vi "WILT.vi"() -> ()   [LabVIEW 2016]
uses:
  Type Definitions/WILT Station Test State Cluster.ctl
  Type Definitions/WILT Dryer Test State.ctl
  Type Definitions/WILT Dryer.ctl
  Type Definitions/WILT Dryer Details.ctl
  Type Definitions/WILT Agilent Channel Definition.ctl
  Type Definitions/WILT DAQ Data.ctl
  Type Definitions/WILT Day Night Cycle Enum.ctl
  Type Definitions/WILT Injection Times.ctl
  Type Definitions/WILT Water Injection Control.ctl
  Utility/Save File/File Setup (Public)/Type Definition/Save File DOE File Path Control.ctl
  Utility/Save File/File Setup (Public)/Type Definition/Save File DOE Data Save Filepaths.ctl
  Type Definitions/WILT Agilent Data Cluster.ctl
  Type Definitions/WILT Summary Data.ctl
  Type Definitions/WILT Water Valve Cluster.ctl
  Type Definitions/WILT Start Button Cluster.ctl
  Type Definitions/WILT Water Valve Test Type.ctl
  Utility/Save File/File Setup (Public)/Type Definition/Save File DOE LabView Program.ctl
  Type Definitions/WILT Switch Search.ctl
  Utility/Save File/Public/Type Definitions/Save File FileName Control.ctl
  <vilib>/Utility/file.llb/Write Delimited Spreadsheet (string).vi
  Globals/WILT Globals Main Program.vi
  Utility/Save File/Save File.lvlib
  Utility/Save File/File Setup.lvlib
panel:
  in  "Final Start Presses":i32=1
  in  "Delay After Cutout (Sec)":dbl=5.0 format="%#_13g"
  out "Agilent Semaphore":T1[](array[typedef])
  out "Version":string
  in  "Agilent Switches":T2[](array[typedef])
  in  "Station Timeout Values (1-56) Seconds":dbl[](array[numeric])
  out "Aisle 4 Location":i32
  out "Aisle 4 Update":T3 {"Night Cycle Count" format="%04d"; "Day Cycle Count" format="%04d"}
  out "Aisle 3 Location":i32
  out "Aisle 3 Update":T3 {"Night Cycle Count" format="%04d"; "Day Cycle Count" format="%04d"}
  out "Aisle 2 Location":i32
  out "Aisle 2 Update":T3 {"Night Cycle Count" format="%04d"; "Day Cycle Count" format="%04d"}
  out "Aisle 1A Location":i32
  out "Aisle 1A Update":T3 {"Night Cycle Count" format="%04d"; "Day Cycle Count" format="%04d"}
  out "Aisle 1 Location":i32
  out "Aisle 1 Update":T3 {"Night Cycle Count" format="%04d"; "Day Cycle Count" format="%04d"}
  out "File Refnums":refnum<file>[](array[refnum])
  out "Agilent Data Out":T6
  in  "Save Rate (Seconds)":i32=1
  in  "Scan Rate (Seconds)":i32=1
  out "New File":bool[](array[boolean])
  out "Waiting For Start":u32(colorbox)=15698688
  out "Watering":u32(colorbox)=15698688
  out "No Com":u32(colorbox)
  out "Running":u32(colorbox)=6618880
  out "Stopped":u32(colorbox)=16776960
  out "Fault":u32(colorbox)=16711680
  out "Unused":u32(colorbox)=7171459
  in  "Debug Tab":enum32{"Page 1", "Page 2", "Page 3"}(tab)
  in  "Reset Start Retry All True":bool
  out "Test State array 2":string[](array[string])
  out "Test State array 3":string[](array[string])
  out "Error Out":errorcluster
  in  "Error In":errorcluster
  in  "Debug 2":bool
  out "Test State array 4":string[](array[string])
  out "UI Runs":i32
  in  "Current Threshold":dbl=0.5 format="%#_13g"
  out "Enable Start Retry Array":bool[](array[boolean])
  out "Agilent Switches Locations":T2[](array[typedef])
  out "Send Restart Every? (Sec)":dbl
  out "Station Test State Cluster 2":T7
  out "Previous Run Statistics":T9[](array[typedef])
  in  "Drying Time (Min)":dbl[](array[numeric])
  out "Uncorrected Agilent Data":dbl[](array[numeric])
  out "Corrected Agilent Data":dbl[](array[numeric])
  out "Exit Signal":bool
  in  "Main Tab":T10(tab)
  in  "Shutdown All Valves":bool
  in  "Reset Start Retry":bool
  in  "Day/Night Cycle":T11
  in  "GUI Aisle 3.":T3[](array[typedef]) {"Night Cycle Count" format="%04d"; "Day Cycle Count" format="%04d"}
  in  "GUI Aisle 1 (SLAT).":T3[](array[typedef]) {"Night Cycle Count" format="%04d"; "Day Cycle Count" format="%04d"}
  in  "GUI Aisle 1A (SLAT).":T3[](array[typedef]) {"Night Cycle Count" format="%04d"; "Day Cycle Count" format="%04d"}
  in  "GUI Aisle 2.":T3[](array[typedef]) {"Night Cycle Count" format="%04d"; "Day Cycle Count" format="%04d"}
  in  "GUI Aisle 4.":T3[](array[typedef]) {"Night Cycle Count" format="%04d"; "Day Cycle Count" format="%04d"}
  in  "ExitProg":bool
  in  "Disable Flood Check":bool
  in  "Valve ON Time (mS)":u32=1000
  in  "Number of ON/OFF Cycles":i32=1
  in  "Test Type":T12
  in  "Start Buttons Cluster":T13
  in  "Water Valves Cluster":T14
  in  "Injection Times":T15
  in  "Agilent Refs":refnum<visa-resource-name>[](array[refnum])=["AGILENT1", "AGILENT2", "AGILENT3", "AGILENT4", "AGILENT5", "AGILENT6", "AGILENT7"]
  out "Initialization Complete":bool
  out "Data Out Array":T6
  in  "File Locations":T17[](array[typedef])
  in  "Station Test State Cluster":T7
  out "Elapsed Time.":dbl format="%<%H:%M:%S>t"
  out "4":T1
  out "3":T1
  out "2":T1
  out "1A":T1
  out "1":T1
  # "Dryer Life Test (WILT)"
  # "Day"
  # "Night"
  # "Day"
  # "Night"
  # "Day"
  # "Night"
  # "Day"
  # "Night"
  # "Day"
  # "Night"
  # "Day"
  # "Night"
  # "Day"
  # "Night"
  # "Day"
  # "Night"
  # "Day"
  # "Night"
  # "Day"
  # "Night"
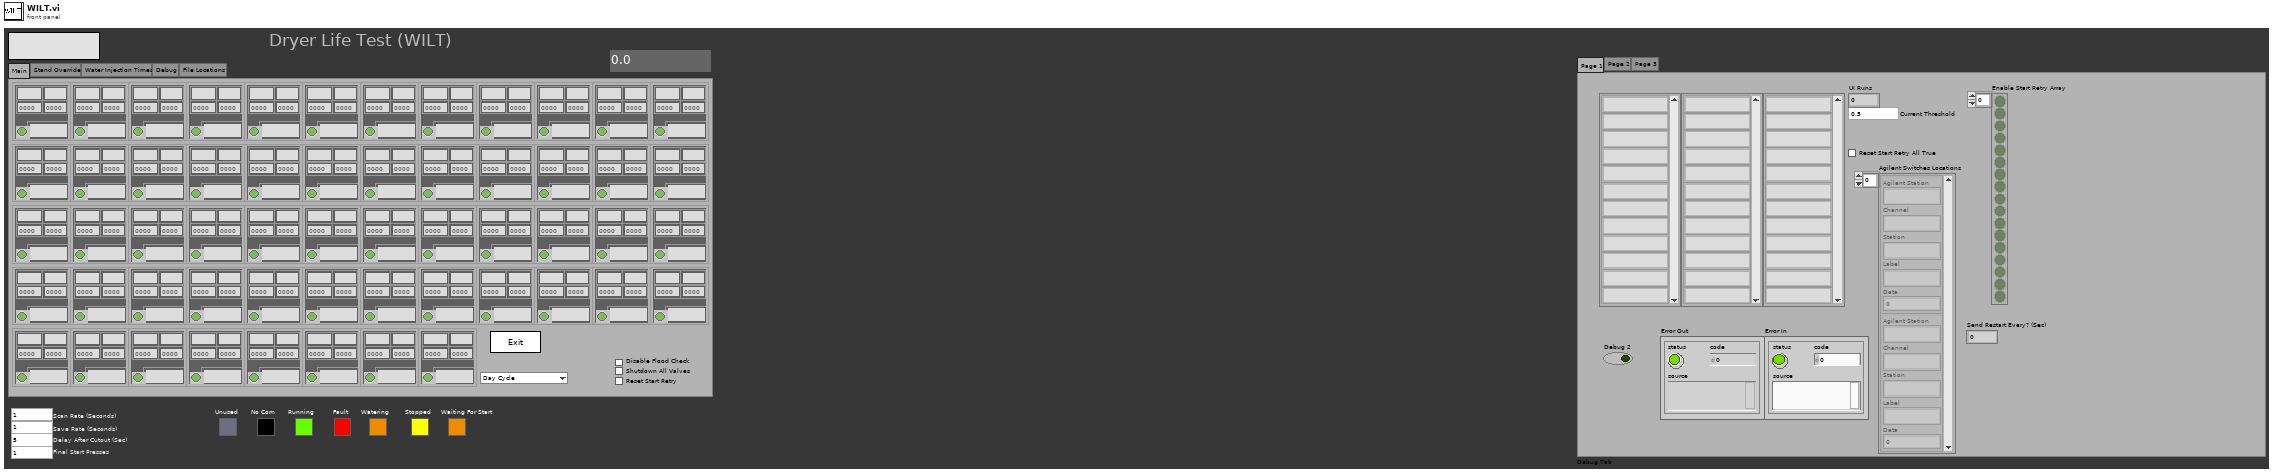
[diagram p1: front panel]
types:
  T1 = typedef "Semaphore RefNum" = refnum<k1>
  T2 = typedef "WILT Agilent Channel Definition.ctl" = cluster{"Channel":string, "Station":string, "Label":string, "Agilent Station":string, "Data":dbl}
  T3 = typedef "WILT Dryer.ctl" = cluster{"Lab ID":string, "Day Cycle Count":i32, "Station Label":string, "Dryer Details":T4, "Status Color":u32, "Invisible Button":bool, "Night Cycle Count":i32, "Station Index":i32, "Cycle Index":string, "Audit Alert":bool, "Agilent Channel Definition":T2, "DAQ Data":T5}
  T4 = typedef "WILT Dryer Details.ctl" = cluster{"Station":string, "Lab ID":string, "TR Number":string}
  T5 = typedef "WILT DAQ Data.ctl" = cluster{"L1 Current":dbl, "L2 Current":dbl, "Temperature  Deg F (TC)":dbl, "Volts":dbl, "Volts (208)":dbl, "SW (208)":dbl}
  T6 = typedef "WILT Agilent Data Cluster.ctl" = T2[]
  T7 = typedef "WILT Station Test State Cluster.ctl" = cluster{"Station Test State 1":T8, "Station Test State 2":T8, "Station Test State 3":T8, "Station Test State 4":T8, "Station Test State 5":T8, "Station Test State 6":T8, "Station Test State 7":T8, "Station Test State 8":T8, "Station Test State 9":T8, "Station Test State 10":T8, "Station Test State 11":T8, "Station Test State 12":T8, "Station Test State 13":T8, "Station Test State 14":T8, "Station Test State 15":T8, "Station Test State 16":T8, "Station Test State 17":T8, "Station Test State 18":T8, "Station Test State 19":T8, "Station Test State 20":T8, "Station Test State 21":T8, "Station Test State 22":T8, "Station Test State 23":T8, "Station Test State 24":T8, "Station Test State 25":T8, "Station Test State 26":T8, "Station Test State 27":T8, "Station Test State 28":T8, "Station Test State 29":T8, "Station Test State 30":T8, "Station Test State 31":T8, "Station Test State 32":T8, "Station Test State 33":T8, "Station Test State 34":T8, "Station Test State 35":T8, "Station Test State 36":T8, "Station Test State 37":T8, "Station Test State 38":T8, "Station Test State 39":T8, "Station Test State 40":T8, "Station Test State 41":T8, "Station Test State 42":T8, "Station Test State 43":T8, "Station Test State 44":T8, "Station Test State 45":T8, "Station Test State 46":T8, "Station Test State 47":T8, "Station Test State 48":T8, "Station Test State 49":T8, "Station Test State 50":T8, "Station Test State 51":T8, "Station Test State 52":T8, "Station Test State 53":T8, "Station Test State 54":T8, "Station Test State 55":T8, "Station Test State 56":T8}
  T8 = typedef "WILT Dryer Test State.ctl" = enum16{"No Serial Number", "Waiting for Dryer To Start", "Drying Clothes", "Water Injection 1 (On)", "Water Injection 1 Timer", "Water Injection 1 (Off)", "Pause Dryer", "Sending Start Stop CMD", "Pause Dryer 2", "Sending Start Stop CMD 2", "Drying Clothes 2", "Water Injection 2 (On)", "Water Injection 2 Timer", "Water Injection 2 (Off)", "Drying Clothes 3", "Cooling Down", "Sending Start Stop CMD 3", "Increment Cycle"}
  T9 = typedef "WILT Summary Data.ctl" = cluster{"Cycle Time (Minutes)":dbl, "L1 Current (Amps)":dbl, "L2 Current (Amps)":dbl, "TC Temperature (Deg F)":dbl, "Voltage (Volts)":dbl, "Voltage-208 (Volts)":dbl, "208V Switch (Ohms)":dbl, "Cycle Number":i32}
  T10 = enum32{"Main", "Stand Override", "Water Injection Times", "Debug", "File Locations"}
  T11 = typedef "WILT Day Night Cycle Enum.ctl" = enum16{"Day Cycle", "Night Cycle", "Day Cycle (No Water)"}
  T12 = typedef "WILT Water Valve Test Type.ctl" = enum16{"Cycle Valve Control", "Full Valve Control"}
  T13 = typedef "WILT Start Button Cluster.ctl" = cluster{"Start Button 21":bool, "Start Button 22":bool, "Start Button 23":bool, "Start Button 24":bool, "Start Button 25":bool, "Start Button 26":bool, "Start Button 27":bool, "Start Button 28":bool, "Start Button 29":bool, "Start Button 30":bool, "Start Button 31":bool, "Start Button 32":bool, "Start Button 33":bool, "Start Button 34":bool, "Start Button 35":bool, "Start Button 36":bool, "Start Button 37":bool, "Start Button 38":bool, "Start Button 39":bool, "Start Button 40":bool, "Start Button 41":bool, "Start Button 42":bool, "Start Button 43":bool, "Start Button 44":bool, "Start Button 12":bool, "Start Button 11":bool, "Start Button 10":bool, "Start Button 9":bool, "Start Button 8":bool, "Start Button 7":bool, "Start Button 6":bool, "Start Button 5":bool, "Start Button 4":bool, "Start Button 3":bool, "Start Button 2":bool, "Start Button 1":bool, "Start Button 20":bool, "Start Button 19":bool, "Start Button 18":bool, "Start Button 17":bool, "Start Button 16":bool, "Start Button 15":bool, "Start Button 14":bool, "Start Button 13":bool, "Start Button 45":bool, "Start Button 46":bool, "Start Button 47":bool, "Start Button 48":bool, "Start Button 49":bool, "Start Button 50":bool, "Start Button 51":bool, "Start Button 52":bool, "Start Button 53":bool, "Start Button 54":bool, "Start Button 55":bool, "Start Button 56":bool}
  T14 = typedef "WILT Water Valve Cluster.ctl" = cluster{"Valve 1":bool, "Valve 2":bool, "Valve 3":bool, "Valve 4":bool, "Valve 5":bool, "Valve 6":bool, "Valve 7":bool, "Valve 8":bool, "Valve 9":bool, "Valve 10":bool, "Valve 11":bool, "Valve 12":bool, "Valve 13":bool, "Valve 14":bool, "Valve 15":bool, "Valve 16":bool, "Valve 17":bool, "Valve 18":bool, "Valve 19":bool, "Valve 20":bool, "Valve 21":bool, "Valve 22":bool, "Valve 23":bool, "Valve 24":bool, "Valve 25":bool, "Valve 26":bool, "Valve 27":bool, "Valve 28":bool, "Valve 29":bool, "Valve 30":bool, "Valve 31":bool, "Valve 32":bool, "Valve 33":bool, "Valve 34":bool, "Valve 35":bool, "Valve 36":bool, "Valve 37":bool, "Valve 38":bool, "Valve 39":bool, "Valve 40":bool, "Valve 41":bool, "Valve 42":bool, "Valve 43":bool, "Valve 44":bool, "Valve 45":bool, "Valve 46":bool, "Valve 47":bool, "Valve 48":bool, "Valve 49":bool, "Valve 50":bool, "Valve 51":bool, "Valve 52":bool, "Valve 53":bool, "Valve 54":bool, "Valve 55":bool, "Valve 56":bool}
  T15 = typedef "WILT Injection Times.ctl" = T16[]
  T16 = typedef "WILT Water Injection Control.ctl" = cluster{"Injection 1 (Seconds)":dbl, "Injection 2 (Seconds)":dbl}
  T17 = typedef "File Setup.lvlib/Save File DOE File Path Control.ctl" = cluster{"General Setup Paths":cluster{"Calibration File Path":path, "DOE Capacity Path":path, "Data Folder Path":path, "RLT Backup Data Path":path, "Tool Base Path":path, "General Startup Config Path":path, "File Save Previous Run Path":path, "File Save Configuration Data Path":path}, "Data File Paths":T18, "New Summary Created":bool, "Check Location Interval (Second)":i32}
  T18 = typedef "File Setup.lvlib/Save File DOE Data Save Filepaths.ctl" = cluster{"Data File Path":path, "Debug File Path":path, "Bus Log Path":path, "Current":path, "Summary":path}
  T19 = typedef "WILT Switch Search.ctl" = string
  T20 = enum32{"invalid app kind", "Development System", "Run Time System", "Student Edition", "Embedded LabVIEW", "Evaluation", "Custom"}
  T21 = typedef "Save File.lvlib/Save File FileName Control.ctl" = cluster{"Debug File DIR":string, "Inverter And MC File DIR":string}
  T22 = enum32{"Invalid", "Standard", "Closed", "Hidden", "Minimized", "Maximized"}
  T23 = typedef "File Setup.lvlib/Save File DOE LabView Program.ctl" = enum16{"No Name Found", "DOE Stand", "Dishwasher Kitchen", "Portable Stand", "HEWH", "Dryer", "Dryer WILT", "HCC", "PRAT", "HEWH RLT", "Refrigeration"}
  T24 = cluster{"Send Restart Every? (Sec)":dbl, "Enable Start Retry Array":bool[], "Agilent Switches":T2[], "States":string, "Core":cluster{"Current VI Reference":refnum<vi>, "Close Panel on Exit?":bool}, "Station Test State Cluster":T7, "GUI Aisle 4.":T3[], "GUI Aisle 3.":T3[], "GUI Aisle 2.":T3[], "GUI Aisle 1A (SLAT).":T3[], "GUI Aisle 1 (SLAT).":T3[], "Agilent Refs":refnum<visa-resource-name>[], "Configuration Startup Directorys":T21, "File Locations":T17[], "Day/Night Cycle Input":T11, "Injection Times Input":T15, "Current Threshold":dbl, "Station Timeout Values (1-56) Seconds":dbl[], "Drying Time (Min)":dbl[]}
  T25 = cluster{"Current VI Reference":refnum<vi>, "Close Panel on Exit?":bool}
  T26 = typedef "Save File.lvlib/Save File Washer.ctl" = cluster{"Appliance Details":T27, "Display Data (RLT)":T33}
  T27 = typedef "File Setup.lvlib/Save File DISH Dishwasher Details.ctl" = cluster{"FileVersionInfo":T28, "Dishwasher Info":cluster{"Open Cup Weight (gm):":dbl, "Auto Cup Weight (gm):":dbl, "Detergent-Dish:":string, "Inlet Temperature-Dish:":string, "Cycle Mode-Dish:":string, "Unit Control-Dish:":string, "Manufacturer-Dish:":string}, "Washer Info":cluster{"Hot Water Temperature (Fahrenheit):":string, "Cold Water Temperature (Fahrenheit):":string, "Capacity (cu.ft):":dbl, "Initial Cloth Weight:":dbl, "Cloth Lot:":i32, "Model Family:":string, "Program Name:":string, "Cycle Selection:":string, "Wash Temperature:":string, "Rinse Temperature:":string, "Load Size:":string}, "File Name Output Array":string[][], "Calibration Output Array":string[][], "Appliance Common":T29, "Water Heater":cluster{"Heating Mode:":string}, "Dryer":cluster{"Heat Setting:":T30, "Washer Water Temperature (60 ± 5°F):":u16, "Water Hardness (PPM):":u16, "Dryness Setting:":T30, "Dryer Type:":string, "Exhaust:":string, "Drying Cycle:":string, "Load Type:":string, "Nominal Load Weight":string, "Dryer Initial IMC Data":T31}}
  T28 = typedef "FileVersionInformation.ctl" = cluster{"FileVersion":string, "ProductName":string, "InternalName":string, "CompanyName":string, "LegalCopyright":string, "FileDescription":string}
  T29 = typedef "DOE Appliance Common.ctl" = cluster{"Engineer:":string, "Model Number:":string, "Serial Number:":string, "Comments:":string, "Station ID:":string, "Technician:":string, "TR Number:":string, "Lab ID:":string, "Voltage:":string, "Water Pressure (PSI):":string, "Test Date:":string, "Computer Name:":string, "IP Address:":string, "Ambient RH:":string, "Frequency:":string, "Build:":string, "Filename:":string, "Test Type:":string, "Load Run #:":i32, "Ambient Temperature (F):":string, "File Path:":path, "Cycles Per Year":u32}
  T30 = typedef "Custom Pallet String.ctl" = string
  T31 = typedef "DPT IMC Data.ctl" = cluster{"Measured IMC (lbs)":dbl, "Actual Initial RMC (%)":dbl, "RMC (Desired %)":dbl, "Bone Dry Wt(lbs)":dbl, "Tolerance(%)":dbl, "Actual Final RMC (%)":dbl, "CEF (lbf/kWh)":dbl, "Minimum Weight (lbf)":dbl, "Average Weight (lbf)":dbl, "Maximum Weight (lbf)":dbl, "Measured IMC In Range?":bool, "Moisture Reduction Factor":dbl, "Field Use Factor":dbl, "Empty Dryer Cold Weigth":dbl, "Energy Standard":T32, "Weight Cloth (lbs)":dbl, "Relative Moisture Content (%)":dbl, "Relative Moisture Content - Avg (%)":dbl}
  T32 = typedef "DOE Dryer Standard.ctl" = enum16{"D2-Automatic Dryer", "D2-Timer Dryer", "D1-Automatic Dryer", "D1-Timer Dryer", "Other"}
  T33 = typedef "Save File Appliance Display.ctl" = cluster{"Status Color":u32, "Serial Number Display":string, "Cycle Count Display":i32, "Station Label Display":string, "Current Run Start Time Display":dbl, "Board ID Display":string, "RPM Display":u32, "Current Display":dbl, "Current Path Display":path, "Saving Display":bool, "Unit Type Display":T34, "Total Time On Display":dbl, "UI Button":bool}
  T34 = typedef "Save File.lvlib/Save File Unit Type.ctl" = enum32{"", "Viper", "Hawk", "2015"}
  T35 = cluster{"Core":cluster{"Current VI Reference":refnum<vi>, "Close Panel on Exit?":bool}, "Agilent Refs":refnum<visa-resource-name>[], "Data Out Array":T6}
  T36 = cluster{"Core":cluster{"Current VI Reference":refnum<vi>, "Close Panel on Exit?":bool}, "First Time Through?":bool[], "File Locations":T17[], "File Refnums":refnum<file>[]}
  T37 = cluster{"File Locations":T17[], "WILT Summary Array":T9[], "Units To Process":bool[]}
  T38 = cluster{"Your Boolean data":bool, "Your string data":string}
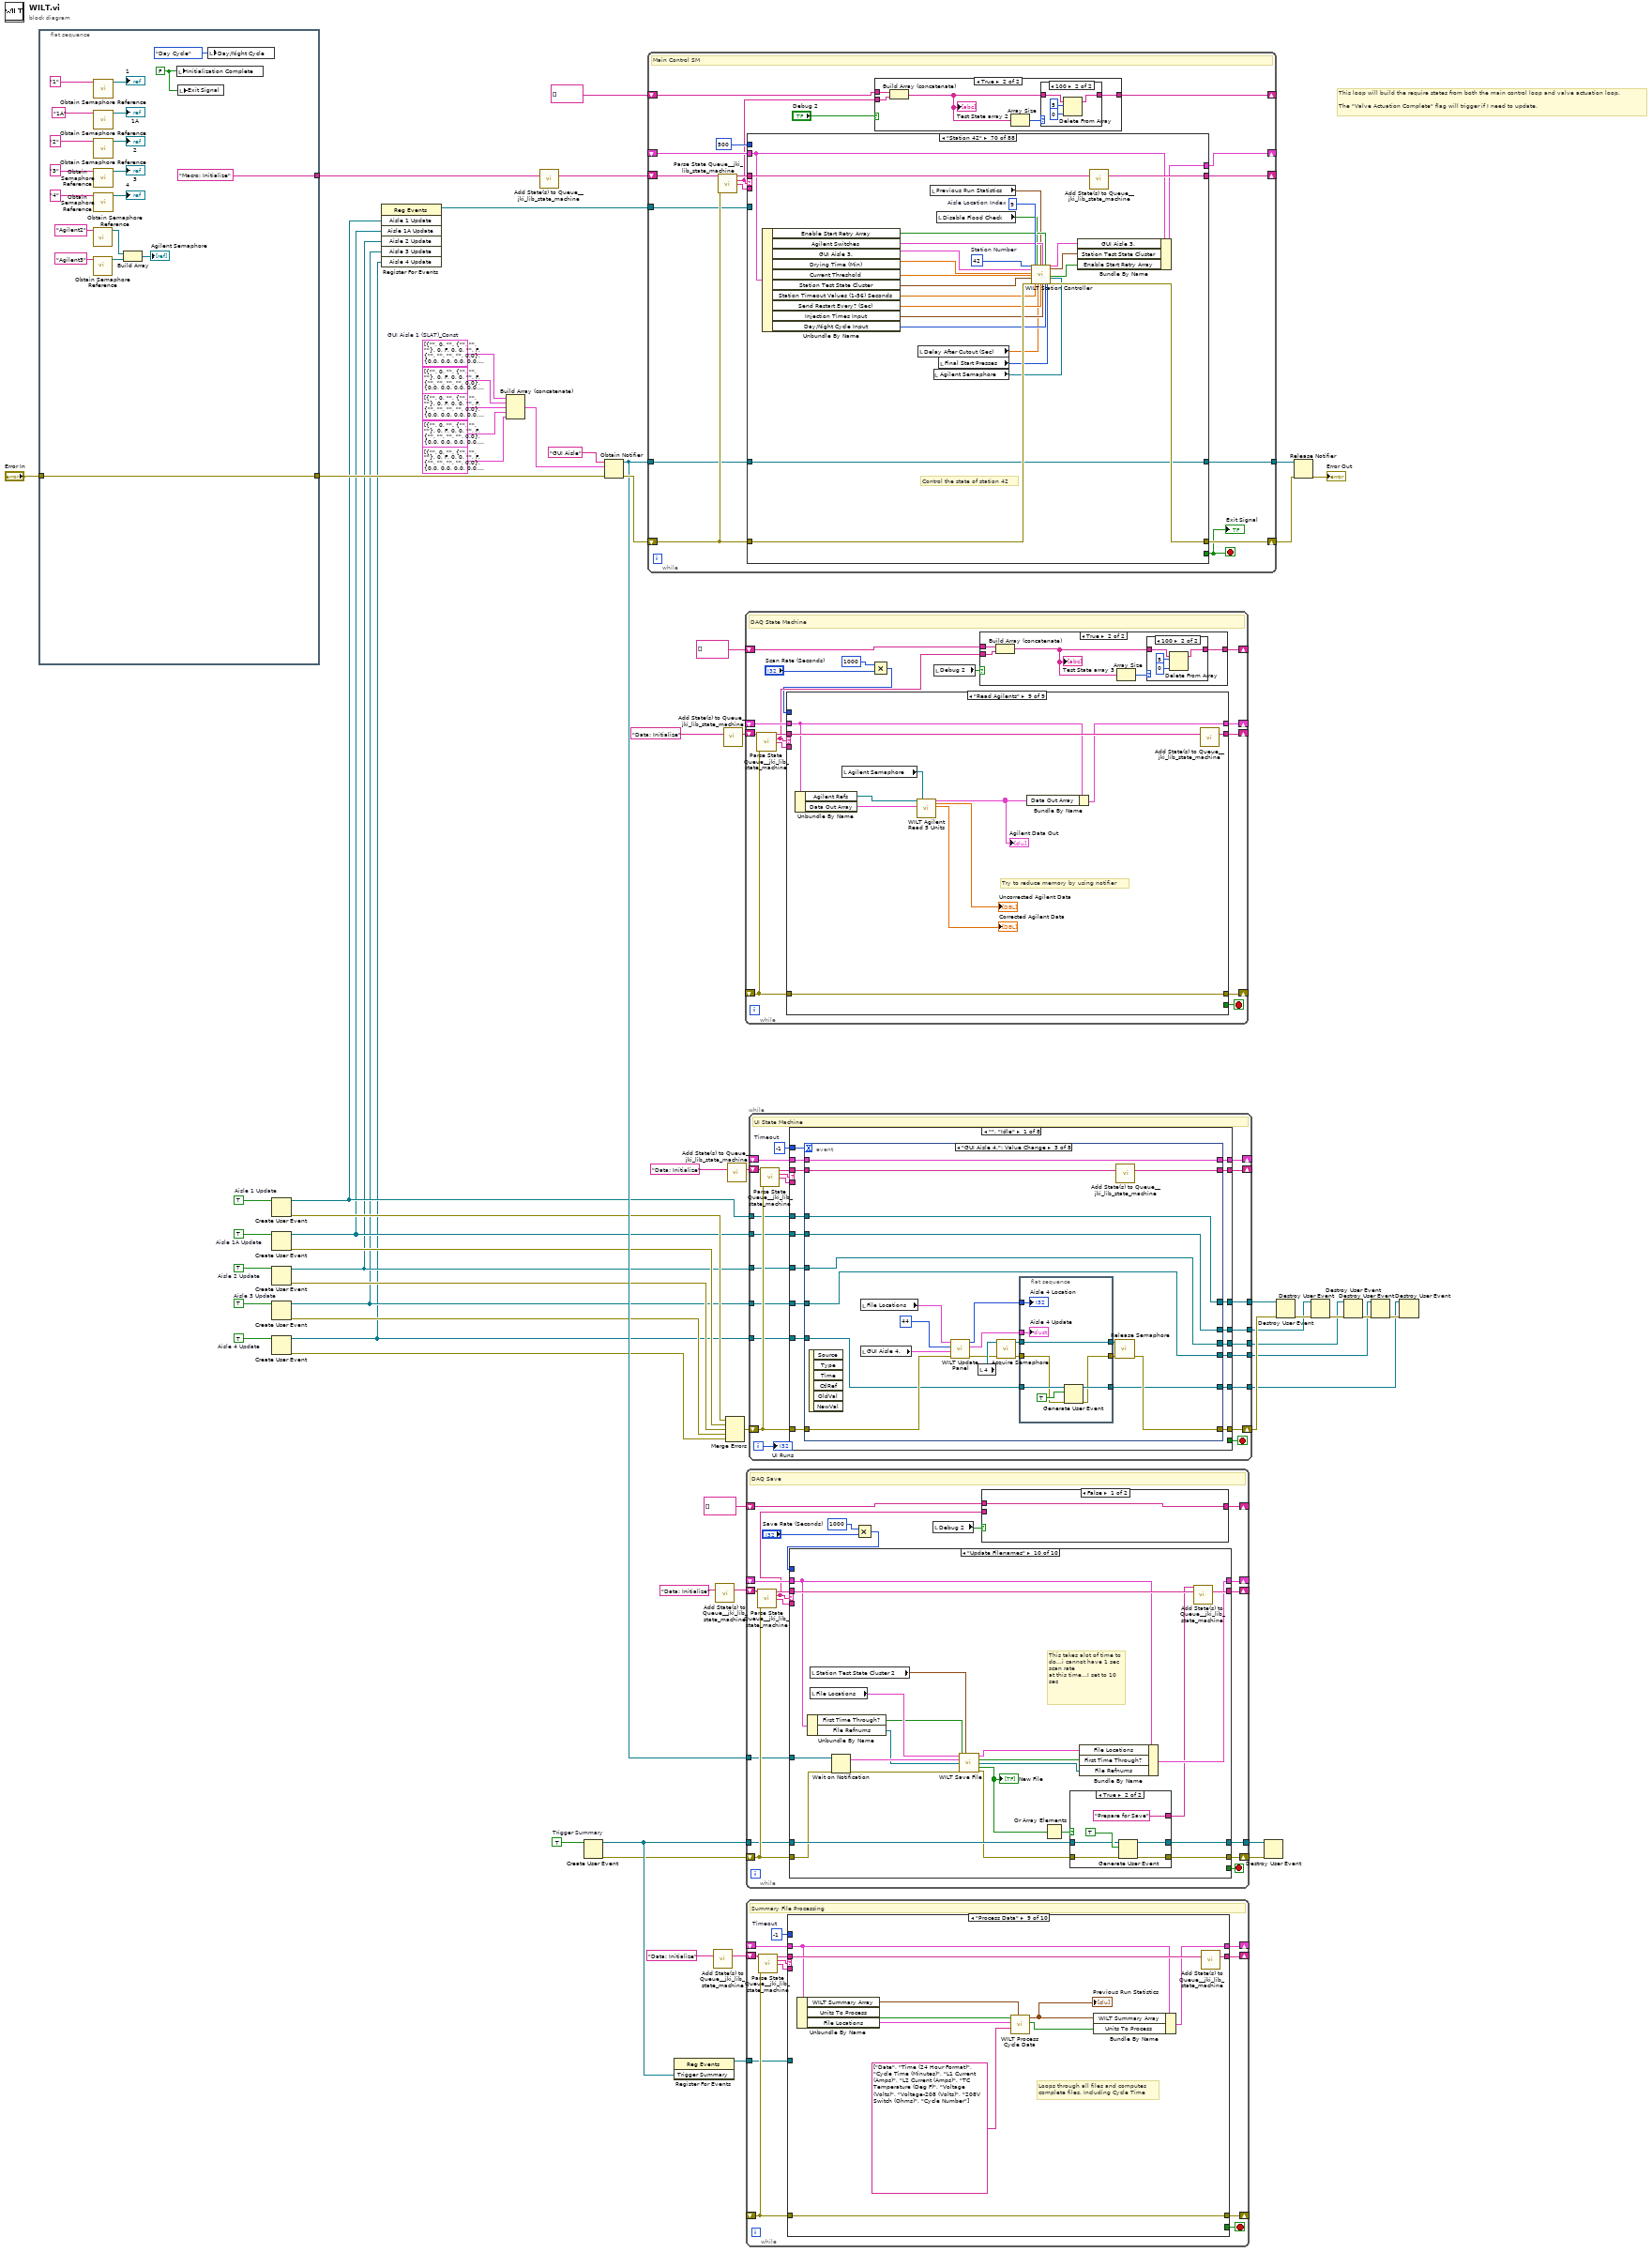
[diagram p0: block diagram]
diagram:
  w24 = TRUE  # Aisle 4 Update
  w25 = TRUE  # Aisle 3 Update
  w26 = TRUE  # Aisle 2 Update
  w27 = TRUE  # Aisle 1A Update
  w28 = TRUE  # Aisle 1 Update
  w39 = T3[] [{"Lab ID"="", "Day Cycle Count"=0, "Station Label"="", "Dryer Details"={"Station"="", "Lab ID"="", "TR Number"=""}, "Status Color"=0, "Invisible Button"=FALSE, "Night Cycle Count"=0, "Station Index"=0, "Cycle Index"="", "Audit Alert"=FALSE, "Agilent Channel Definition"={"Channel"="", "Station"="", "Label"="", "Agilent Station"="", "Data"=0.0}, "DAQ Data"={"L1 Current"=0.0, "L2 Current"=0.0, "Temperature  Deg F (TC)"=0.0, "Volts"=0.0, "Volts (208)"=0.0, "SW (208)"=0.0}}, {"Lab ID"="", "Day Cycle Count"=0, "Station Label"="", "Dryer Details"={"Station"="", "Lab ID"="", "TR Number"=""}, "Status Color"=0, "Invisible Button"=FALSE, "Night Cycle Count"=0, "Station Index"=0, "Cycle Index"="", "Audit Alert"=FALSE, "Agilent Channel Definition"={"Channel"="", "Station"="", "Label"="", "Agilent Station"="", "Data"=0.0}, "DAQ Data"={"L1 Current"=0.0, "L2 Current"=0.0, "Temperature  Deg F (TC)"=0.0, "Volts"=0.0, "Volts (208)"=0.0, "SW (208)"=0.0}}, {"Lab ID"="", "Day Cycle Count"=0, "Station Label"="", "Dryer Details"={"Station"="", "Lab ID"="", "TR Number"=""}, "Status Color"=0, "Invisible Button"=FALSE, "Night Cycle Count"=0, "Station Index"=0, "Cycle Index"="", "Audit Alert"=FALSE, "Agilent Channel Definition"={"Channel"="", "Station"="", "Label"="", "Agilent Station"="", "Data"=0.0}, "DAQ Data"={"L1 Current"=0.0, "L2 Current"=0.0, "Temperature  Deg F (TC)"=0.0, "Volts"=0.0, "Volts (208)"=0.0, "SW (208)"=0.0}}, {"Lab ID"="", "Day Cycle Count"=0, "Station Label"="", "Dryer Details"={"Station"="", "Lab ID"="", "TR Number"=""}, "Status Color"=0, "Invisible Button"=FALSE, "Night Cycle Count"=0, "Station Index"=0, "Cycle Index"="", "Audit Alert"=FALSE, "Agilent Channel Definition"={"Channel"="", "Station"="", "Label"="", "Agilent Station"="", "Data"=0.0}, "DAQ Data"={"L1 Current"=0.0, "L2 Current"=0.0, "Temperature  Deg F (TC)"=0.0, "Volts"=0.0, "Volts (208)"=0.0, "SW (208)"=0.0}}, {"Lab ID"="", "Day Cycle Count"=0, "Station Label"="", "Dryer Details"={"Station"="", "Lab ID"="", "TR Number"=""}, "Status Color"=0, "Invisible Button"=FALSE, "Night Cycle Count"=0, "Station Index"=0, "Cycle Index"="", "Audit Alert"=FALSE, "Agilent Channel Definition"={"Channel"="", "Station"="", "Label"="", "Agilent Station"="", "Data"=0.0}, "DAQ Data"={"L1 Current"=0.0, "L2 Current"=0.0, "Temperature  Deg F (TC)"=0.0, "Volts"=0.0, "Volts (208)"=0.0, "SW (208)"=0.0}}, {"Lab ID"="", "Day Cycle Count"=0, "Station Label"="", "Dryer Details"={"Station"="", "Lab ID"="", "TR Number"=""}, "Status Color"=0, "Invisible Button"=FALSE, "Night Cycle Count"=0, "Station Index"=0, "Cycle Index"="", "Audit Alert"=FALSE, "Agilent Channel Definition"={"Channel"="", "Station"="", "Label"="", "Agilent Station"="", "Data"=0.0}, "DAQ Data"={"L1 Current"=0.0, "L2 Current"=0.0, "Temperature  Deg F (TC)"=0.0, "Volts"=0.0, "Volts (208)"=0.0, "SW (208)"=0.0}}, {"Lab ID"="", "Day Cycle Count"=0, "Station Label"="", "Dryer Details"={"Station"="", "Lab ID"="", "TR Number"=""}, "Status Color"=0, "Invisible Button"=FALSE, "Night Cycle Count"=0, "Station Index"=0, "Cycle Index"="", "Audit Alert"=FALSE, "Agilent Channel Definition"={"Channel"="", "Station"="", "Label"="", "Agilent Station"="", "Data"=0.0}, "DAQ Data"={"L1 Current"=0.0, "L2 Current"=0.0, "Temperature  Deg F (TC)"=0.0, "Volts"=0.0, "Volts (208)"=0.0, "SW (208)"=0.0}}, {"Lab ID"="", "Day Cycle Count"=0, "Station Label"="", "Dryer Details"={"Station"="", "Lab ID"="", "TR Number"=""}, "Status Color"=0, "Invisible Button"=FALSE, "Night Cycle Count"=0, "Station Index"=0, "Cycle Index"="", "Audit Alert"=FALSE, "Agilent Channel Definition"={"Channel"="", "Station"="", "Label"="", "Agilent Station"="", "Data"=0.0}, "DAQ Data"={"L1 Current"=0.0, "L2 Current"=0.0, "Temperature  Deg F (TC)"=0.0, "Volts"=0.0, "Volts (208)"=0.0, "SW (208)"=0.0}}, {"Lab ID"="", "Day Cycle Count"=0, "Station Label"="", "Dryer Details"={"Station"="", "Lab ID"="", "TR Number"=""}, "Status Color"=0, "Invisible Button"=FALSE, "Night Cycle Count"=0, "Station Index"=0, "Cycle Index"="", "Audit Alert"=FALSE, "Agilent Channel Definition"={"Channel"="", "Station"="", "Label"="", "Agilent Station"="", "Data"=0.0}, "DAQ Data"={"L1 Current"=0.0, "L2 Current"=0.0, "Temperature  Deg F (TC)"=0.0, "Volts"=0.0, "Volts (208)"=0.0, "SW (208)"=0.0}}, {"Lab ID"="", "Day Cycle Count"=0, "Station Label"="", "Dryer Details"={"Station"="", "Lab ID"="", "TR Number"=""}, "Status Color"=0, "Invisible Button"=FALSE, "Night Cycle Count"=0, "Station Index"=0, "Cycle Index"="", "Audit Alert"=FALSE, "Agilent Channel Definition"={"Channel"="", "Station"="", "Label"="", "Agilent Station"="", "Data"=0.0}, "DAQ Data"={"L1 Current"=0.0, "L2 Current"=0.0, "Temperature  Deg F (TC)"=0.0, "Volts"=0.0, "Volts (208)"=0.0, "SW (208)"=0.0}}, {"Lab ID"="", "Day Cycle Count"=0, "Station Label"="", "Dryer Details"={"Station"="", "Lab ID"="", "TR Number"=""}, "Status Color"=0, "Invisible Button"=FALSE, "Night Cycle Count"=0, "Station Index"=0, "Cycle Index"="", "Audit Alert"=FALSE, "Agilent Channel Definition"={"Channel"="", "Station"="", "Label"="", "Agilent Station"="", "Data"=0.0}, "DAQ Data"={"L1 Current"=0.0, "L2 Current"=0.0, "Temperature  Deg F (TC)"=0.0, "Volts"=0.0, "Volts (208)"=0.0, "SW (208)"=0.0}}, {"Lab ID"="", "Day Cycle Count"=0, "Station Label"="", "Dryer Details"={"Station"="", "Lab ID"="", "TR Number"=""}, "Status Color"=0, "Invisible Button"=FALSE, "Night Cycle Count"=0, "Station Index"=0, "Cycle Index"="", "Audit Alert"=FALSE, "Agilent Channel Definition"={"Channel"="", "Station"="", "Label"="", "Agilent Station"="", "Data"=0.0}, "DAQ Data"={"L1 Current"=0.0, "L2 Current"=0.0, "Temperature  Deg F (TC)"=0.0, "Volts"=0.0, "Volts (208)"=0.0, "SW (208)"=0.0}}]  # GUI Aisle 1 (SLAT)_Const
  w46 = TRUE  # Trigger Summary
  # "This loop will build the require states from both the main control loop and valve actuation loop.\n\nThe \"Valve Actuation Complete\" flag will trigger if I need to update."
  n1 = flat-sequence {
    tunnel: ["Macro: Initialize"] -> w59
    tunnel: [w76] -> w34
    tunnel: "Error In" -> [w76]
    frame #0 {
      w78 = FALSE ("Initialization Complete")
      n2 = call <vilib>:"Obtain Semaphore Reference.vi"("name (unnamed)"="Agilent2") -> ("semaphore"=w63:T1)  [unwired: 4 in, 2 out]
      n3 = call <vilib>:"Obtain Semaphore Reference.vi"("name (unnamed)"="Agilent3") -> ("semaphore"=w62:T1)  [unwired: 4 in, 2 out]
      n4 = call <vilib>:"Obtain Semaphore Reference.vi"("name (unnamed)"="1") -> ("semaphore"=→"1":T1)  [unwired: 4 in, 2 out]
      n5 = call <vilib>:"Obtain Semaphore Reference.vi"("name (unnamed)"="1A") -> ("semaphore"=→"1A":T1)  [unwired: 4 in, 2 out]
      n6 = call <vilib>:"Obtain Semaphore Reference.vi"("name (unnamed)"="2") -> ("semaphore"=→"2":T1)  [unwired: 4 in, 2 out]
      n7 = call <vilib>:"Obtain Semaphore Reference.vi"("name (unnamed)"="3") -> ("semaphore"=→"3":T1)  [unwired: 4 in, 2 out]
      n8 = call <vilib>:"Obtain Semaphore Reference.vi"("name (unnamed)"="4") -> ("semaphore"=→"4":T1)  [unwired: 4 in, 2 out]
      n9 = Build Array(w63, w62) -> (→"Agilent Semaphore":T1[])
      n10 = local write "Initialization Complete"(w78) -> ()
      n11 = local write "Exit Signal"(w78) -> ()
      n12 = local write "Day/Night Cycle"(WILT_Day_Night_Cycle_Enum."Day Cycle" ("Day/Night Cycle")) -> ()
    }
  }
  n13 = Create User Event(user event datatype=w28) -> (user event=w7:refnum<user-event>, error out=w23:errorcluster)  [unwired: 1 in]
  n14 = Create User Event(user event datatype=w27) -> (user event=w6:refnum<user-event>, error out=w22:errorcluster)  [unwired: 1 in]
  n15 = Create User Event(user event datatype=w26) -> (user event=w5:refnum<user-event>, error out=w21:errorcluster)  [unwired: 1 in]
  n16 = Create User Event(user event datatype=w25) -> (user event=w4:refnum<user-event>, error out=w20:errorcluster)  [unwired: 1 in]
  n17 = Create User Event(user event datatype=w24) -> (user event=w3:refnum<user-event>, error out=w19:errorcluster)  [unwired: 1 in]
  n18 = register-events(w7, w6, w5, w4, w3) -> (reference out=w2:refnum<event-registration>)  [unwired: 2 in, 1 out]
  n19 = Build Array (concatenate)(w39, T3[] [{"Lab ID"="", "Day Cycle Count"=0, "Station Label"="", "Dryer Details"={"Station"="", "Lab ID"="", "TR Number"=""}, "Status Color"=0, "Invisible Button"=FALSE, "Night Cycle Count"=0, "Station Index"=0, "Cycle Index"="", "Audit Alert"=FALSE, "Agilent Channel Definition"={"Channel"="", "Station"="", "Label"="", "Agilent Station"="", "Data"=0.0}, "DAQ Data"={"L1 Current"=0.0, "L2 Current"=0.0, "Temperature  Deg F (TC)"=0.0, "Volts"=0.0, "Volts (208)"=0.0, "SW (208)"=0.0}}, {"Lab ID"="", "Day Cycle Count"=0, "Station Label"="", "Dryer Details"={"Station"="", "Lab ID"="", "TR Number"=""}, "Status Color"=0, "Invisible Button"=FALSE, "Night Cycle Count"=0, "Station Index"=0, "Cycle Index"="", "Audit Alert"=FALSE, "Agilent Channel Definition"={"Channel"="", "Station"="", "Label"="", "Agilent Station"="", "Data"=0.0}, "DAQ Data"={"L1 Current"=0.0, "L2 Current"=0.0, "Temperature  Deg F (TC)"=0.0, "Volts"=0.0, "Volts (208)"=0.0, "SW (208)"=0.0}}, {"Lab ID"="", "Day Cycle Count"=0, "Station Label"="", "Dryer Details"={"Station"="", "Lab ID"="", "TR Number"=""}, "Status Color"=0, "Invisible Button"=FALSE, "Night Cycle Count"=0, "Station Index"=0, "Cycle Index"="", "Audit Alert"=FALSE, "Agilent Channel Definition"={"Channel"="", "Station"="", "Label"="", "Agilent Station"="", "Data"=0.0}, "DAQ Data"={"L1 Current"=0.0, "L2 Current"=0.0, "Temperature  Deg F (TC)"=0.0, "Volts"=0.0, "Volts (208)"=0.0, "SW (208)"=0.0}}, {"Lab ID"="", "Day Cycle Count"=0, "Station Label"="", "Dryer Details"={"Station"="", "Lab ID"="", "TR Number"=""}, "Status Color"=0, "Invisible Button"=FALSE, "Night Cycle Count"=0, "Station Index"=0, "Cycle Index"="", "Audit Alert"=FALSE, "Agilent Channel Definition"={"Channel"="", "Station"="", "Label"="", "Agilent Station"="", "Data"=0.0}, "DAQ Data"={"L1 Current"=0.0, "L2 Current"=0.0, "Temperature  Deg F (TC)"=0.0, "Volts"=0.0, "Volts (208)"=0.0, "SW (208)"=0.0}}, {"Lab ID"="", "Day Cycle Count"=0, "Station Label"="", "Dryer Details"={"Station"="", "Lab ID"="", "TR Number"=""}, "Status Color"=0, "Invisible Button"=FALSE, "Night Cycle Count"=0, "Station Index"=0, "Cycle Index"="", "Audit Alert"=FALSE, "Agilent Channel Definition"={"Channel"="", "Station"="", "Label"="", "Agilent Station"="", "Data"=0.0}, "DAQ Data"={"L1 Current"=0.0, "L2 Current"=0.0, "Temperature  Deg F (TC)"=0.0, "Volts"=0.0, "Volts (208)"=0.0, "SW (208)"=0.0}}, {"Lab ID"="", "Day Cycle Count"=0, "Station Label"="", "Dryer Details"={"Station"="", "Lab ID"="", "TR Number"=""}, "Status Color"=0, "Invisible Button"=FALSE, "Night Cycle Count"=0, "Station Index"=0, "Cycle Index"="", "Audit Alert"=FALSE, "Agilent Channel Definition"={"Channel"="", "Station"="", "Label"="", "Agilent Station"="", "Data"=0.0}, "DAQ Data"={"L1 Current"=0.0, "L2 Current"=0.0, "Temperature  Deg F (TC)"=0.0, "Volts"=0.0, "Volts (208)"=0.0, "SW (208)"=0.0}}, {"Lab ID"="", "Day Cycle Count"=0, "Station Label"="", "Dryer Details"={"Station"="", "Lab ID"="", "TR Number"=""}, "Status Color"=0, "Invisible Button"=FALSE, "Night Cycle Count"=0, "Station Index"=0, "Cycle Index"="", "Audit Alert"=FALSE, "Agilent Channel Definition"={"Channel"="", "Station"="", "Label"="", "Agilent Station"="", "Data"=0.0}, "DAQ Data"={"L1 Current"=0.0, "L2 Current"=0.0, "Temperature  Deg F (TC)"=0.0, "Volts"=0.0, "Volts (208)"=0.0, "SW (208)"=0.0}}, {"Lab ID"="", "Day Cycle Count"=0, "Station Label"="", "Dryer Details"={"Station"="", "Lab ID"="", "TR Number"=""}, "Status Color"=0, "Invisible Button"=FALSE, "Night Cycle Count"=0, "Station Index"=0, "Cycle Index"="", "Audit Alert"=FALSE, "Agilent Channel Definition"={"Channel"="", "Station"="", "Label"="", "Agilent Station"="", "Data"=0.0}, "DAQ Data"={"L1 Current"=0.0, "L2 Current"=0.0, "Temperature  Deg F (TC)"=0.0, "Volts"=0.0, "Volts (208)"=0.0, "SW (208)"=0.0}}] ("GUI Aisle 1A (SLAT)_Const"), T3[] [{"Lab ID"="", "Day Cycle Count"=0, "Station Label"="", "Dryer Details"={"Station"="", "Lab ID"="", "TR Number"=""}, "Status Color"=0, "Invisible Button"=FALSE, "Night Cycle Count"=0, "Station Index"=0, "Cycle Index"="", "Audit Alert"=FALSE, "Agilent Channel Definition"={"Channel"="", "Station"="", "Label"="", "Agilent Station"="", "Data"=0.0}, "DAQ Data"={"L1 Current"=0.0, "L2 Current"=0.0, "Temperature  Deg F (TC)"=0.0, "Volts"=0.0, "Volts (208)"=0.0, "SW (208)"=0.0}}, {"Lab ID"="", "Day Cycle Count"=0, "Station Label"="", "Dryer Details"={"Station"="", "Lab ID"="", "TR Number"=""}, "Status Color"=0, "Invisible Button"=FALSE, "Night Cycle Count"=0, "Station Index"=0, "Cycle Index"="", "Audit Alert"=FALSE, "Agilent Channel Definition"={"Channel"="", "Station"="", "Label"="", "Agilent Station"="", "Data"=0.0}, "DAQ Data"={"L1 Current"=0.0, "L2 Current"=0.0, "Temperature  Deg F (TC)"=0.0, "Volts"=0.0, "Volts (208)"=0.0, "SW (208)"=0.0}}, {"Lab ID"="", "Day Cycle Count"=0, "Station Label"="", "Dryer Details"={"Station"="", "Lab ID"="", "TR Number"=""}, "Status Color"=0, "Invisible Button"=FALSE, "Night Cycle Count"=0, "Station Index"=0, "Cycle Index"="", "Audit Alert"=FALSE, "Agilent Channel Definition"={"Channel"="", "Station"="", "Label"="", "Agilent Station"="", "Data"=0.0}, "DAQ Data"={"L1 Current"=0.0, "L2 Current"=0.0, "Temperature  Deg F (TC)"=0.0, "Volts"=0.0, "Volts (208)"=0.0, "SW (208)"=0.0}}, {"Lab ID"="", "Day Cycle Count"=0, "Station Label"="", "Dryer Details"={"Station"="", "Lab ID"="", "TR Number"=""}, "Status Color"=0, "Invisible Button"=FALSE, "Night Cycle Count"=0, "Station Index"=0, "Cycle Index"="", "Audit Alert"=FALSE, "Agilent Channel Definition"={"Channel"="", "Station"="", "Label"="", "Agilent Station"="", "Data"=0.0}, "DAQ Data"={"L1 Current"=0.0, "L2 Current"=0.0, "Temperature  Deg F (TC)"=0.0, "Volts"=0.0, "Volts (208)"=0.0, "SW (208)"=0.0}}, {"Lab ID"="", "Day Cycle Count"=0, "Station Label"="", "Dryer Details"={"Station"="", "Lab ID"="", "TR Number"=""}, "Status Color"=0, "Invisible Button"=FALSE, "Night Cycle Count"=0, "Station Index"=0, "Cycle Index"="", "Audit Alert"=FALSE, "Agilent Channel Definition"={"Channel"="", "Station"="", "Label"="", "Agilent Station"="", "Data"=0.0}, "DAQ Data"={"L1 Current"=0.0, "L2 Current"=0.0, "Temperature  Deg F (TC)"=0.0, "Volts"=0.0, "Volts (208)"=0.0, "SW (208)"=0.0}}, {"Lab ID"="", "Day Cycle Count"=0, "Station Label"="", "Dryer Details"={"Station"="", "Lab ID"="", "TR Number"=""}, "Status Color"=0, "Invisible Button"=FALSE, "Night Cycle Count"=0, "Station Index"=0, "Cycle Index"="", "Audit Alert"=FALSE, "Agilent Channel Definition"={"Channel"="", "Station"="", "Label"="", "Agilent Station"="", "Data"=0.0}, "DAQ Data"={"L1 Current"=0.0, "L2 Current"=0.0, "Temperature  Deg F (TC)"=0.0, "Volts"=0.0, "Volts (208)"=0.0, "SW (208)"=0.0}}, {"Lab ID"="", "Day Cycle Count"=0, "Station Label"="", "Dryer Details"={"Station"="", "Lab ID"="", "TR Number"=""}, "Status Color"=0, "Invisible Button"=FALSE, "Night Cycle Count"=0, "Station Index"=0, "Cycle Index"="", "Audit Alert"=FALSE, "Agilent Channel Definition"={"Channel"="", "Station"="", "Label"="", "Agilent Station"="", "Data"=0.0}, "DAQ Data"={"L1 Current"=0.0, "L2 Current"=0.0, "Temperature  Deg F (TC)"=0.0, "Volts"=0.0, "Volts (208)"=0.0, "SW (208)"=0.0}}, {"Lab ID"="", "Day Cycle Count"=0, "Station Label"="", "Dryer Details"={"Station"="", "Lab ID"="", "TR Number"=""}, "Status Color"=0, "Invisible Button"=FALSE, "Night Cycle Count"=0, "Station Index"=0, "Cycle Index"="", "Audit Alert"=FALSE, "Agilent Channel Definition"={"Channel"="", "Station"="", "Label"="", "Agilent Station"="", "Data"=0.0}, "DAQ Data"={"L1 Current"=0.0, "L2 Current"=0.0, "Temperature  Deg F (TC)"=0.0, "Volts"=0.0, "Volts (208)"=0.0, "SW (208)"=0.0}}, {"Lab ID"="", "Day Cycle Count"=0, "Station Label"="", "Dryer Details"={"Station"="", "Lab ID"="", "TR Number"=""}, "Status Color"=0, "Invisible Button"=FALSE, "Night Cycle Count"=0, "Station Index"=0, "Cycle Index"="", "Audit Alert"=FALSE, "Agilent Channel Definition"={"Channel"="", "Station"="", "Label"="", "Agilent Station"="", "Data"=0.0}, "DAQ Data"={"L1 Current"=0.0, "L2 Current"=0.0, "Temperature  Deg F (TC)"=0.0, "Volts"=0.0, "Volts (208)"=0.0, "SW (208)"=0.0}}, {"Lab ID"="", "Day Cycle Count"=0, "Station Label"="", "Dryer Details"={"Station"="", "Lab ID"="", "TR Number"=""}, "Status Color"=0, "Invisible Button"=FALSE, "Night Cycle Count"=0, "Station Index"=0, "Cycle Index"="", "Audit Alert"=FALSE, "Agilent Channel Definition"={"Channel"="", "Station"="", "Label"="", "Agilent Station"="", "Data"=0.0}, "DAQ Data"={"L1 Current"=0.0, "L2 Current"=0.0, "Temperature  Deg F (TC)"=0.0, "Volts"=0.0, "Volts (208)"=0.0, "SW (208)"=0.0}}, {"Lab ID"="", "Day Cycle Count"=0, "Station Label"="", "Dryer Details"={"Station"="", "Lab ID"="", "TR Number"=""}, "Status Color"=0, "Invisible Button"=FALSE, "Night Cycle Count"=0, "Station Index"=0, "Cycle Index"="", "Audit Alert"=FALSE, "Agilent Channel Definition"={"Channel"="", "Station"="", "Label"="", "Agilent Station"="", "Data"=0.0}, "DAQ Data"={"L1 Current"=0.0, "L2 Current"=0.0, "Temperature  Deg F (TC)"=0.0, "Volts"=0.0, "Volts (208)"=0.0, "SW (208)"=0.0}}, {"Lab ID"="", "Day Cycle Count"=0, "Station Label"="", "Dryer Details"={"Station"="", "Lab ID"="", "TR Number"=""}, "Status Color"=0, "Invisible Button"=FALSE, "Night Cycle Count"=0, "Station Index"=0, "Cycle Index"="", "Audit Alert"=FALSE, "Agilent Channel Definition"={"Channel"="", "Station"="", "Label"="", "Agilent Station"="", "Data"=0.0}, "DAQ Data"={"L1 Current"=0.0, "L2 Current"=0.0, "Temperature  Deg F (TC)"=0.0, "Volts"=0.0, "Volts (208)"=0.0, "SW (208)"=0.0}}] ("GUI Aisle 2_Const"), T3[] [{"Lab ID"="", "Day Cycle Count"=0, "Station Label"="", "Dryer Details"={"Station"="", "Lab ID"="", "TR Number"=""}, "Status Color"=0, "Invisible Button"=FALSE, "Night Cycle Count"=0, "Station Index"=0, "Cycle Index"="", "Audit Alert"=FALSE, "Agilent Channel Definition"={"Channel"="", "Station"="", "Label"="", "Agilent Station"="", "Data"=0.0}, "DAQ Data"={"L1 Current"=0.0, "L2 Current"=0.0, "Temperature  Deg F (TC)"=0.0, "Volts"=0.0, "Volts (208)"=0.0, "SW (208)"=0.0}}, {"Lab ID"="", "Day Cycle Count"=0, "Station Label"="", "Dryer Details"={"Station"="", "Lab ID"="", "TR Number"=""}, "Status Color"=0, "Invisible Button"=FALSE, "Night Cycle Count"=0, "Station Index"=0, "Cycle Index"="", "Audit Alert"=FALSE, "Agilent Channel Definition"={"Channel"="", "Station"="", "Label"="", "Agilent Station"="", "Data"=0.0}, "DAQ Data"={"L1 Current"=0.0, "L2 Current"=0.0, "Temperature  Deg F (TC)"=0.0, "Volts"=0.0, "Volts (208)"=0.0, "SW (208)"=0.0}}, {"Lab ID"="", "Day Cycle Count"=0, "Station Label"="", "Dryer Details"={"Station"="", "Lab ID"="", "TR Number"=""}, "Status Color"=0, "Invisible Button"=FALSE, "Night Cycle Count"=0, "Station Index"=0, "Cycle Index"="", "Audit Alert"=FALSE, "Agilent Channel Definition"={"Channel"="", "Station"="", "Label"="", "Agilent Station"="", "Data"=0.0}, "DAQ Data"={"L1 Current"=0.0, "L2 Current"=0.0, "Temperature  Deg F (TC)"=0.0, "Volts"=0.0, "Volts (208)"=0.0, "SW (208)"=0.0}}, {"Lab ID"="", "Day Cycle Count"=0, "Station Label"="", "Dryer Details"={"Station"="", "Lab ID"="", "TR Number"=""}, "Status Color"=0, "Invisible Button"=FALSE, "Night Cycle Count"=0, "Station Index"=0, "Cycle Index"="", "Audit Alert"=FALSE, "Agilent Channel Definition"={"Channel"="", "Station"="", "Label"="", "Agilent Station"="", "Data"=0.0}, "DAQ Data"={"L1 Current"=0.0, "L2 Current"=0.0, "Temperature  Deg F (TC)"=0.0, "Volts"=0.0, "Volts (208)"=0.0, "SW (208)"=0.0}}, {"Lab ID"="", "Day Cycle Count"=0, "Station Label"="", "Dryer Details"={"Station"="", "Lab ID"="", "TR Number"=""}, "Status Color"=0, "Invisible Button"=FALSE, "Night Cycle Count"=0, "Station Index"=0, "Cycle Index"="", "Audit Alert"=FALSE, "Agilent Channel Definition"={"Channel"="", "Station"="", "Label"="", "Agilent Station"="", "Data"=0.0}, "DAQ Data"={"L1 Current"=0.0, "L2 Current"=0.0, "Temperature  Deg F (TC)"=0.0, "Volts"=0.0, "Volts (208)"=0.0, "SW (208)"=0.0}}, {"Lab ID"="", "Day Cycle Count"=0, "Station Label"="", "Dryer Details"={"Station"="", "Lab ID"="", "TR Number"=""}, "Status Color"=0, "Invisible Button"=FALSE, "Night Cycle Count"=0, "Station Index"=0, "Cycle Index"="", "Audit Alert"=FALSE, "Agilent Channel Definition"={"Channel"="", "Station"="", "Label"="", "Agilent Station"="", "Data"=0.0}, "DAQ Data"={"L1 Current"=0.0, "L2 Current"=0.0, "Temperature  Deg F (TC)"=0.0, "Volts"=0.0, "Volts (208)"=0.0, "SW (208)"=0.0}}, {"Lab ID"="", "Day Cycle Count"=0, "Station Label"="", "Dryer Details"={"Station"="", "Lab ID"="", "TR Number"=""}, "Status Color"=0, "Invisible Button"=FALSE, "Night Cycle Count"=0, "Station Index"=0, "Cycle Index"="", "Audit Alert"=FALSE, "Agilent Channel Definition"={"Channel"="", "Station"="", "Label"="", "Agilent Station"="", "Data"=0.0}, "DAQ Data"={"L1 Current"=0.0, "L2 Current"=0.0, "Temperature  Deg F (TC)"=0.0, "Volts"=0.0, "Volts (208)"=0.0, "SW (208)"=0.0}}, {"Lab ID"="", "Day Cycle Count"=0, "Station Label"="", "Dryer Details"={"Station"="", "Lab ID"="", "TR Number"=""}, "Status Color"=0, "Invisible Button"=FALSE, "Night Cycle Count"=0, "Station Index"=0, "Cycle Index"="", "Audit Alert"=FALSE, "Agilent Channel Definition"={"Channel"="", "Station"="", "Label"="", "Agilent Station"="", "Data"=0.0}, "DAQ Data"={"L1 Current"=0.0, "L2 Current"=0.0, "Temperature  Deg F (TC)"=0.0, "Volts"=0.0, "Volts (208)"=0.0, "SW (208)"=0.0}}, {"Lab ID"="", "Day Cycle Count"=0, "Station Label"="", "Dryer Details"={"Station"="", "Lab ID"="", "TR Number"=""}, "Status Color"=0, "Invisible Button"=FALSE, "Night Cycle Count"=0, "Station Index"=0, "Cycle Index"="", "Audit Alert"=FALSE, "Agilent Channel Definition"={"Channel"="", "Station"="", "Label"="", "Agilent Station"="", "Data"=0.0}, "DAQ Data"={"L1 Current"=0.0, "L2 Current"=0.0, "Temperature  Deg F (TC)"=0.0, "Volts"=0.0, "Volts (208)"=0.0, "SW (208)"=0.0}}, {"Lab ID"="", "Day Cycle Count"=0, "Station Label"="", "Dryer Details"={"Station"="", "Lab ID"="", "TR Number"=""}, "Status Color"=0, "Invisible Button"=FALSE, "Night Cycle Count"=0, "Station Index"=0, "Cycle Index"="", "Audit Alert"=FALSE, "Agilent Channel Definition"={"Channel"="", "Station"="", "Label"="", "Agilent Station"="", "Data"=0.0}, "DAQ Data"={"L1 Current"=0.0, "L2 Current"=0.0, "Temperature  Deg F (TC)"=0.0, "Volts"=0.0, "Volts (208)"=0.0, "SW (208)"=0.0}}, {"Lab ID"="", "Day Cycle Count"=0, "Station Label"="", "Dryer Details"={"Station"="", "Lab ID"="", "TR Number"=""}, "Status Color"=0, "Invisible Button"=FALSE, "Night Cycle Count"=0, "Station Index"=0, "Cycle Index"="", "Audit Alert"=FALSE, "Agilent Channel Definition"={"Channel"="", "Station"="", "Label"="", "Agilent Station"="", "Data"=0.0}, "DAQ Data"={"L1 Current"=0.0, "L2 Current"=0.0, "Temperature  Deg F (TC)"=0.0, "Volts"=0.0, "Volts (208)"=0.0, "SW (208)"=0.0}}, {"Lab ID"="", "Day Cycle Count"=0, "Station Label"="", "Dryer Details"={"Station"="", "Lab ID"="", "TR Number"=""}, "Status Color"=0, "Invisible Button"=FALSE, "Night Cycle Count"=0, "Station Index"=0, "Cycle Index"="", "Audit Alert"=FALSE, "Agilent Channel Definition"={"Channel"="", "Station"="", "Label"="", "Agilent Station"="", "Data"=0.0}, "DAQ Data"={"L1 Current"=0.0, "L2 Current"=0.0, "Temperature  Deg F (TC)"=0.0, "Volts"=0.0, "Volts (208)"=0.0, "SW (208)"=0.0}}] ("GUI Aisle 3_Const"), T3[] [{"Lab ID"="", "Day Cycle Count"=0, "Station Label"="", "Dryer Details"={"Station"="", "Lab ID"="", "TR Number"=""}, "Status Color"=0, "Invisible Button"=FALSE, "Night Cycle Count"=0, "Station Index"=0, "Cycle Index"="", "Audit Alert"=FALSE, "Agilent Channel Definition"={"Channel"="", "Station"="", "Label"="", "Agilent Station"="", "Data"=0.0}, "DAQ Data"={"L1 Current"=0.0, "L2 Current"=0.0, "Temperature  Deg F (TC)"=0.0, "Volts"=0.0, "Volts (208)"=0.0, "SW (208)"=0.0}}, {"Lab ID"="", "Day Cycle Count"=0, "Station Label"="", "Dryer Details"={"Station"="", "Lab ID"="", "TR Number"=""}, "Status Color"=0, "Invisible Button"=FALSE, "Night Cycle Count"=0, "Station Index"=0, "Cycle Index"="", "Audit Alert"=FALSE, "Agilent Channel Definition"={"Channel"="", "Station"="", "Label"="", "Agilent Station"="", "Data"=0.0}, "DAQ Data"={"L1 Current"=0.0, "L2 Current"=0.0, "Temperature  Deg F (TC)"=0.0, "Volts"=0.0, "Volts (208)"=0.0, "SW (208)"=0.0}}, {"Lab ID"="", "Day Cycle Count"=0, "Station Label"="", "Dryer Details"={"Station"="", "Lab ID"="", "TR Number"=""}, "Status Color"=0, "Invisible Button"=FALSE, "Night Cycle Count"=0, "Station Index"=0, "Cycle Index"="", "Audit Alert"=FALSE, "Agilent Channel Definition"={"Channel"="", "Station"="", "Label"="", "Agilent Station"="", "Data"=0.0}, "DAQ Data"={"L1 Current"=0.0, "L2 Current"=0.0, "Temperature  Deg F (TC)"=0.0, "Volts"=0.0, "Volts (208)"=0.0, "SW (208)"=0.0}}, {"Lab ID"="", "Day Cycle Count"=0, "Station Label"="", "Dryer Details"={"Station"="", "Lab ID"="", "TR Number"=""}, "Status Color"=0, "Invisible Button"=FALSE, "Night Cycle Count"=0, "Station Index"=0, "Cycle Index"="", "Audit Alert"=FALSE, "Agilent Channel Definition"={"Channel"="", "Station"="", "Label"="", "Agilent Station"="", "Data"=0.0}, "DAQ Data"={"L1 Current"=0.0, "L2 Current"=0.0, "Temperature  Deg F (TC)"=0.0, "Volts"=0.0, "Volts (208)"=0.0, "SW (208)"=0.0}}, {"Lab ID"="", "Day Cycle Count"=0, "Station Label"="", "Dryer Details"={"Station"="", "Lab ID"="", "TR Number"=""}, "Status Color"=0, "Invisible Button"=FALSE, "Night Cycle Count"=0, "Station Index"=0, "Cycle Index"="", "Audit Alert"=FALSE, "Agilent Channel Definition"={"Channel"="", "Station"="", "Label"="", "Agilent Station"="", "Data"=0.0}, "DAQ Data"={"L1 Current"=0.0, "L2 Current"=0.0, "Temperature  Deg F (TC)"=0.0, "Volts"=0.0, "Volts (208)"=0.0, "SW (208)"=0.0}}, {"Lab ID"="", "Day Cycle Count"=0, "Station Label"="", "Dryer Details"={"Station"="", "Lab ID"="", "TR Number"=""}, "Status Color"=0, "Invisible Button"=FALSE, "Night Cycle Count"=0, "Station Index"=0, "Cycle Index"="", "Audit Alert"=FALSE, "Agilent Channel Definition"={"Channel"="", "Station"="", "Label"="", "Agilent Station"="", "Data"=0.0}, "DAQ Data"={"L1 Current"=0.0, "L2 Current"=0.0, "Temperature  Deg F (TC)"=0.0, "Volts"=0.0, "Volts (208)"=0.0, "SW (208)"=0.0}}, {"Lab ID"="", "Day Cycle Count"=0, "Station Label"="", "Dryer Details"={"Station"="", "Lab ID"="", "TR Number"=""}, "Status Color"=0, "Invisible Button"=FALSE, "Night Cycle Count"=0, "Station Index"=0, "Cycle Index"="", "Audit Alert"=FALSE, "Agilent Channel Definition"={"Channel"="", "Station"="", "Label"="", "Agilent Station"="", "Data"=0.0}, "DAQ Data"={"L1 Current"=0.0, "L2 Current"=0.0, "Temperature  Deg F (TC)"=0.0, "Volts"=0.0, "Volts (208)"=0.0, "SW (208)"=0.0}}, {"Lab ID"="", "Day Cycle Count"=0, "Station Label"="", "Dryer Details"={"Station"="", "Lab ID"="", "TR Number"=""}, "Status Color"=0, "Invisible Button"=FALSE, "Night Cycle Count"=0, "Station Index"=0, "Cycle Index"="", "Audit Alert"=FALSE, "Agilent Channel Definition"={"Channel"="", "Station"="", "Label"="", "Agilent Station"="", "Data"=0.0}, "DAQ Data"={"L1 Current"=0.0, "L2 Current"=0.0, "Temperature  Deg F (TC)"=0.0, "Volts"=0.0, "Volts (208)"=0.0, "SW (208)"=0.0}}, {"Lab ID"="", "Day Cycle Count"=0, "Station Label"="", "Dryer Details"={"Station"="", "Lab ID"="", "TR Number"=""}, "Status Color"=0, "Invisible Button"=FALSE, "Night Cycle Count"=0, "Station Index"=0, "Cycle Index"="", "Audit Alert"=FALSE, "Agilent Channel Definition"={"Channel"="", "Station"="", "Label"="", "Agilent Station"="", "Data"=0.0}, "DAQ Data"={"L1 Current"=0.0, "L2 Current"=0.0, "Temperature  Deg F (TC)"=0.0, "Volts"=0.0, "Volts (208)"=0.0, "SW (208)"=0.0}}, {"Lab ID"="", "Day Cycle Count"=0, "Station Label"="", "Dryer Details"={"Station"="", "Lab ID"="", "TR Number"=""}, "Status Color"=0, "Invisible Button"=FALSE, "Night Cycle Count"=0, "Station Index"=0, "Cycle Index"="", "Audit Alert"=FALSE, "Agilent Channel Definition"={"Channel"="", "Station"="", "Label"="", "Agilent Station"="", "Data"=0.0}, "DAQ Data"={"L1 Current"=0.0, "L2 Current"=0.0, 
